vi "Build Map from Page GUIDs to Page VIs.vi"() -> (3 "page map GUID to VI ref":map{string, refnum<vi>}(c390))   [LabVIEW 2020, in "Ballard MIL-STD-1553 System Explorer.lvlib" / "Implementation.lvlib" / "System Explorer Dispatcher.lvclass"]
uses:
  System Explorer Dispatcher.lvclass
  System Explorer/Pages/Status.vi
  Implementation.lvlib
  Scripting/Constants.vi
  Scripting/Ballard MIL-STD-1553 Scripting.lvlib
  System Explorer/Pages/Configuration Files.vi
  System Explorer/Pages/Parameter.vi
  System Explorer/Pages/Trigger Channel.vi
  System Explorer/Pages/Subaddress.vi
  System Explorer/Pages/Message.vi
  System Explorer/Pages/Acyclic Frames.vi
  System Explorer/Pages/Remote Terminal.vi
  System Explorer/Pages/Bus Controller.vi
  System Explorer/Pages/Status Section.vi
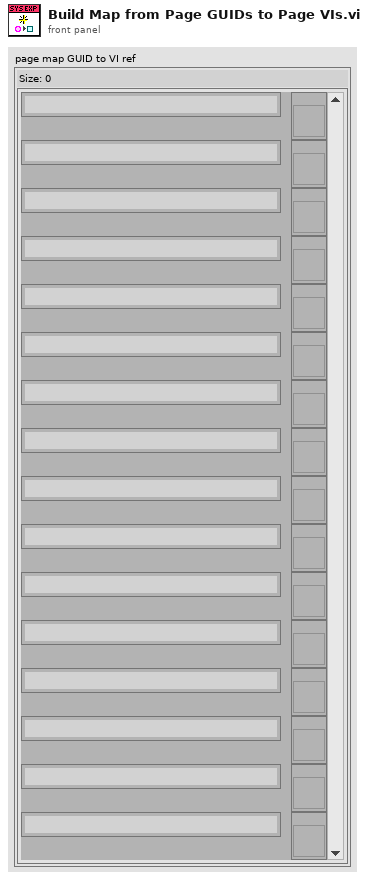
[diagram p1: front panel]
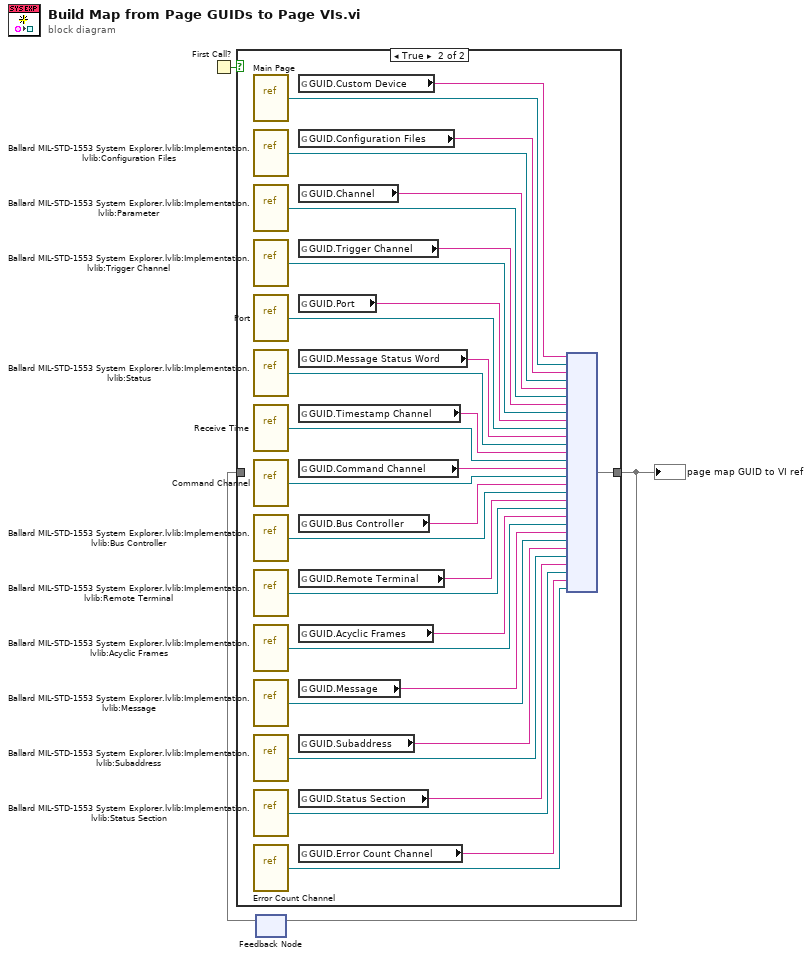
[diagram p0: block diagram]
diagram:
  n1 = First Call?() -> (First Call?: T/F=w1:bool)
  n2 = feedback #1() -> (w2:map{string, refnum<vi>})  [unwired: 1 in]
  n3 = case shown="True" w1 {
    tunnel: [w4 w35] -> w3
    tunnel: w2 -> [w4 _]
    frame False {
    }
    frame True {
      n4 = vi-ref "Main Page.vi"() -> (w34:refnum<vi>)
      n5 = vi-ref "Ballard MIL-STD-1553 System Explorer.lvlib:Implementation.lvlib:Configuration Files.vi"() -> (w32:refnum<vi>)
      n6 = vi-ref "Ballard MIL-STD-1553 System Explorer.lvlib:Implementation.lvlib:Parameter.vi"() -> (w29:refnum<vi>)
      n7 = vi-ref "Ballard MIL-STD-1553 System Explorer.lvlib:Implementation.lvlib:Trigger Channel.vi"() -> (w27:refnum<vi>)
      n8 = vi-ref "Port.vi"() -> (w25:refnum<vi>)
      n9 = vi-ref "Ballard MIL-STD-1553 System Explorer.lvlib:Implementation.lvlib:Status.vi"() -> (w23:refnum<vi>)
      n10 = vi-ref "Receive Time.vi"() -> (w21:refnum<vi>)
      n11 = vi-ref "Command Channel.vi"() -> (w19:refnum<vi>)
      n12 = vi-ref "Ballard MIL-STD-1553 System Explorer.lvlib:Implementation.lvlib:Bus Controller.vi"() -> (w17:refnum<vi>)
      n13 = vi-ref "Ballard MIL-STD-1553 System Explorer.lvlib:Implementation.lvlib:Remote Terminal.vi"() -> (w15:refnum<vi>)
      n14 = vi-ref "Ballard MIL-STD-1553 System Explorer.lvlib:Implementation.lvlib:Acyclic Frames.vi"() -> (w13:refnum<vi>)
      n15 = vi-ref "Ballard MIL-STD-1553 System Explorer.lvlib:Implementation.lvlib:Message.vi"() -> (w11:refnum<vi>)
      n16 = vi-ref "Ballard MIL-STD-1553 System Explorer.lvlib:Implementation.lvlib:Subaddress.vi"() -> (w9:refnum<vi>)
      n17 = vi-ref "Ballard MIL-STD-1553 System Explorer.lvlib:Implementation.lvlib:Status Section.vi"() -> (w7:refnum<vi>)
      n18 = vi-ref "Error Count Channel.vi"() -> (w5:refnum<vi>)
      n19 = global read "Constants.vi" "GUID.Custom Device"() -> (w33:string)
      n20 = global read "Constants.vi" "GUID.Configuration Files"() -> (w31:string)
      n21 = global read "Constants.vi" "GUID.Channel"() -> (w30:string)
      n22 = global read "Constants.vi" "GUID.Trigger Channel"() -> (w28:string)
      n23 = global read "Constants.vi" "GUID.Port"() -> (w26:string)
      n24 = global read "Constants.vi" "GUID.Message Status Word"() -> (w24:string)
      n25 = global read "Constants.vi" "GUID.Timestamp Channel"() -> (w22:string)
      n26 = global read "Constants.vi" "GUID.Command Channel"() -> (w20:string)
      n27 = global read "Constants.vi" "GUID.Bus Controller"() -> (w18:string)
      n28 = global read "Constants.vi" "GUID.Remote Terminal"() -> (w16:string)
      n29 = global read "Constants.vi" "GUID.Acyclic Frames"() -> (w14:string)
      n30 = global read "Constants.vi" "GUID.Message"() -> (w12:string)
      n31 = global read "Constants.vi" "GUID.Subaddress"() -> (w10:string)
      n32 = global read "Constants.vi" "GUID.Status Section"() -> (w8:string)
      n33 = global read "Constants.vi" "GUID.Error Count Channel"() -> (w6:string)
      n34 = node(w33, w34, w31, w32, w30, w29, w28, w27, w26, w25, w24, w23, w22, w21, w20, w19, w18, w17, w16, w15, w14, w13, w12, w11, w10, w9, w8, w7, w6, w5) -> (w35:map{string, refnum<vi>})
    }
  }
  "page map GUID to VI ref" <- w3
  n35 = feedback-in #1(w3) -> ()
